vi "main.vi"() -> ()   [LabVIEW 2020]
uses:
  <vilib>/DAQmx/read.llb/DAQmx Read (Analog 1D DBL 1Chan NSamp).vi
  <vilib>/Analysis/baseanly.llb/Mean (DBL).vi
  <vilib>/Utility/file.llb/Write Delimited Spreadsheet (string).vi
  <vilib>/DAQmx/create/channels.llb/DAQmx Create Channel (AI-Current-Basic).vi
  <vilib>/DAQmx/configure/timing.llb/DAQmx Timing (Sample Clock).vi
  <vilib>/DAQmx/create/channels.llb/DAQmx Create Channel (AI-Voltage-Basic).vi
  <vilib>/Utility/file.llb/Write Delimited Spreadsheet (DBL).vi
  <vilib>/DAQmx/miscellaneous.llb/DAQmx Fill In Error Info.vi
  sub_vi/Timing.llb/getRelativeTime(Host).vi
  <vilib>/Analysis/NI_AALBase.lvlib
  sub_vi/Timing.llb/Timing.lvlib
  sub_vi/PlotGraph.llb/GraphPlot.lvlib
panel:
  out "period(hz)":dbl(knob) scale=0.0..30.0
  out "ElapseTime":string
  out "power_value":dbl format="%0.2f"
  in  "FileName":string="power"
  out "power_praph":cluster{dbl[], dbl[]}(graph)
  out "VI_graph":cluster{dbl[], dbl[]}[](graph)
  out "enable_channel":bool
  out "enable_channel":bool
  in  "stop":bool
  out "ampere_value":dbl format="%0.2f"
  out "voltage_value":dbl format="%0.2f"
  out "ampere_graph":dbl[](graph)
  out "voltage_graph":dbl[](graph)
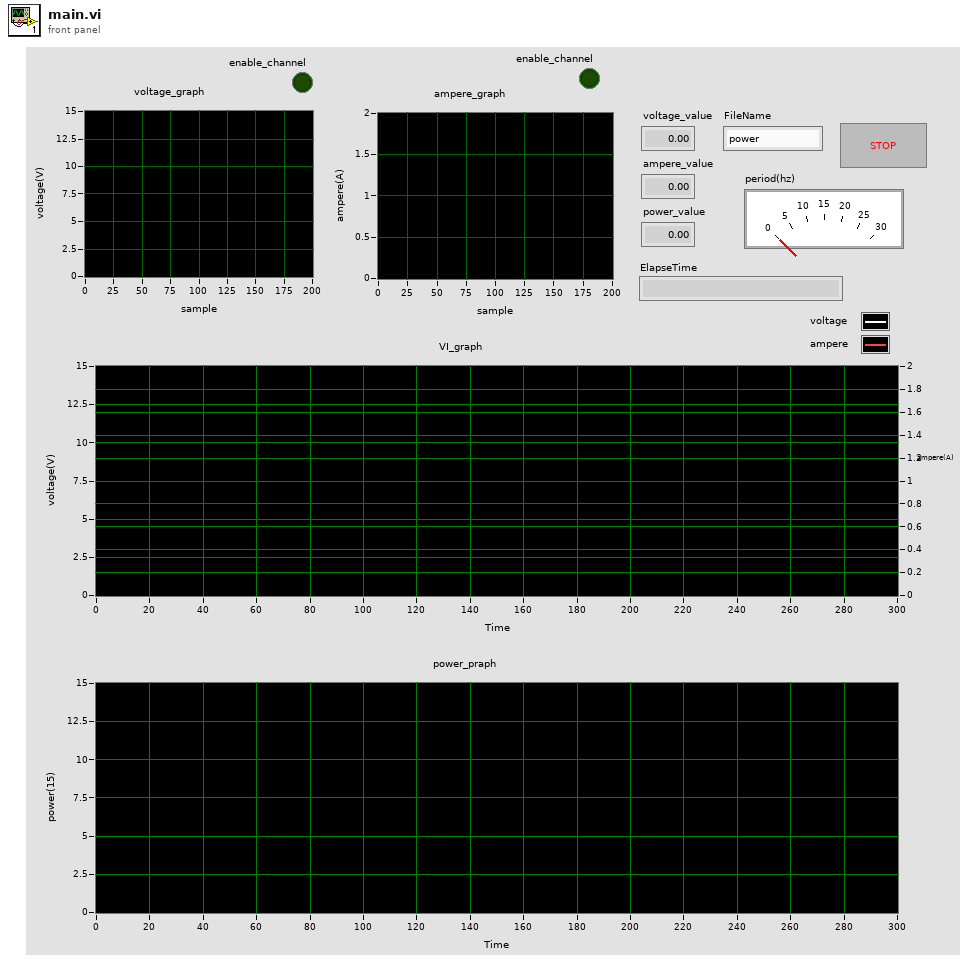
[diagram p1: front panel]
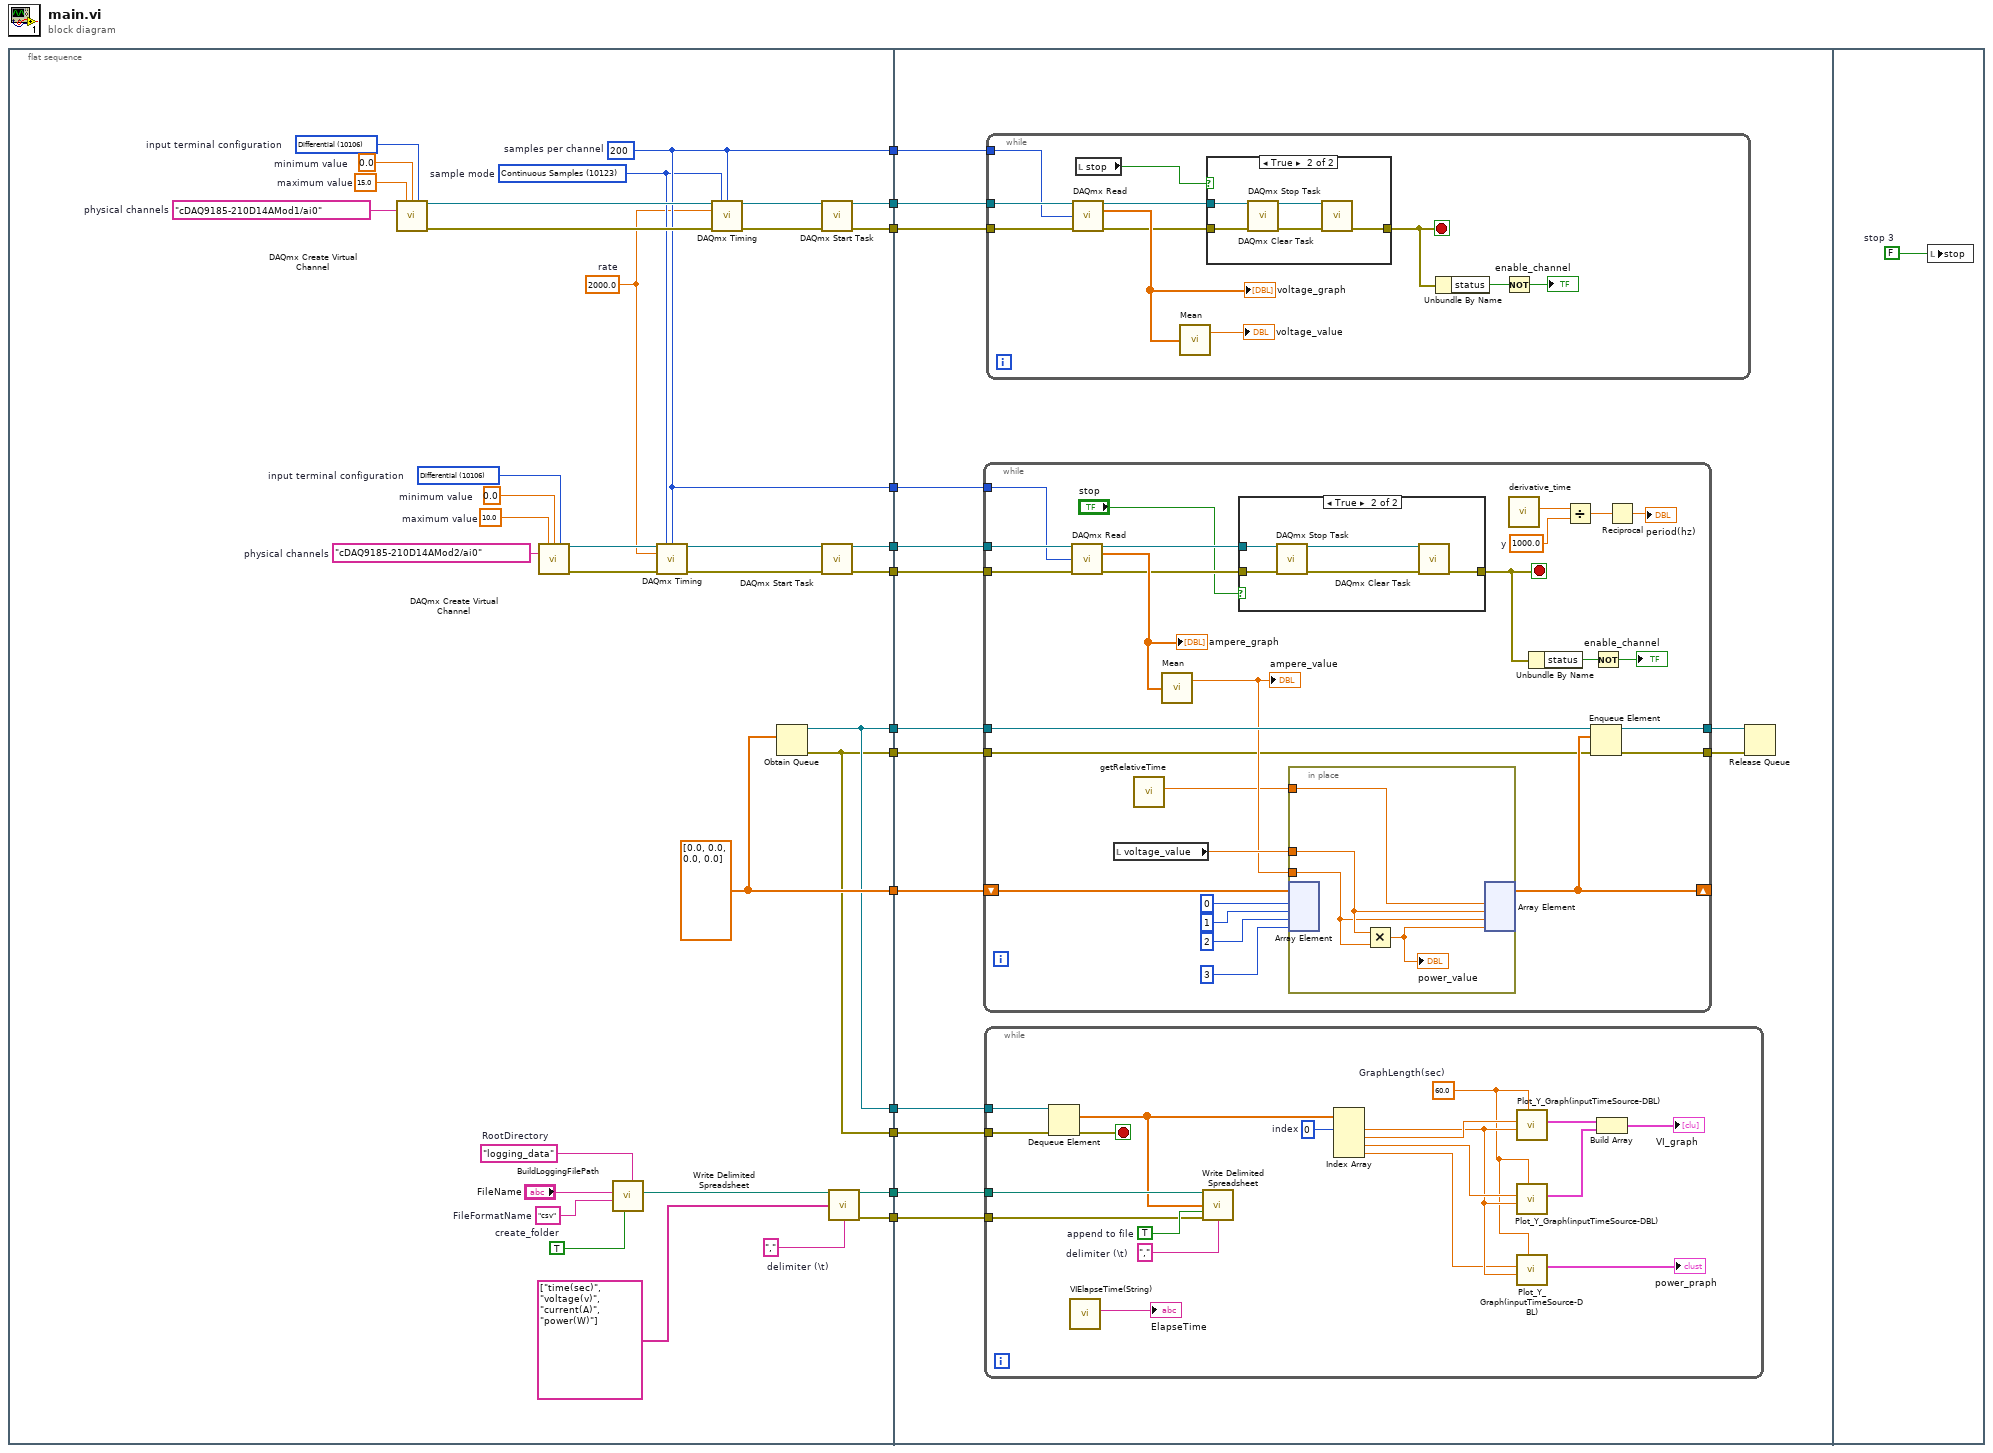
[diagram p0: block diagram]
diagram:
  n1 = flat-sequence {
    tunnel: [w44] -> w13
    tunnel: [w40] -> w12
    tunnel: [w35] -> w11
    tunnel: [w34] -> w10
    tunnel: [w30] -> w9
    tunnel: [w30] -> w8
    tunnel: [w32] -> w7
    tunnel: [w33] -> w6
    tunnel: [w31] -> w5
    tunnel: [w32] -> w4
    tunnel: [w31] -> w3
    tunnel: [w20] -> w2
    tunnel: [w18] -> w1
    tunnel: w13 -> [w63]
    tunnel: w12 -> [w62]
    tunnel: w11 -> [w60]
    tunnel: w10 -> [w59]
    tunnel: w9 -> [w58]
    tunnel: w8 -> [w61]
    tunnel: w7 -> [w57]
    tunnel: w6 -> [w56]
    tunnel: w5 -> [w55]
    tunnel: w4 -> [w54]
    tunnel: w3 -> [w53]
    tunnel: w2 -> [w52]
    tunnel: w1 -> [w51]
    frame #0 {
      w14 = 15.0  # maximum value
      w15 = 0.0  # minimum value
      w16 = 10.0  # maximum value
      w17 = 0.0  # minimum value
      w19 = ","  # delimiter (\t)
      w23 = TRUE  # create_folder
      w24 = "logging_data"  # RootDirectory
      w25 = "csv"  # FileFormatName
      w27 = 10106 items=["Default"=-1, "RSE"=10083, "NRSE"=10078, "Differential"=10106, "Pseudodifferential"=12529]  # input terminal configuration
      w33 = dbl[] [0.0, 0.0, 0.0, 0.0]
      w30 = 200  # samples per channel
      w28 = 2000.0  # rate
      w29 = 10123 items=["Finite Samples"=10178, "Continuous Samples"=10123, "Hardware Timed Single Point"=12522]  # sample mode
      w45 = 10106 items=["default"=-1, "RSE"=10083, "NRSE"=10078, "Differential"=10106, "Pseudodifferential"=12529]  # input terminal configuration
      w47 = tag "cDAQ9185-210D14AMod2/ai0"  # physical channels
      w48 = tag "cDAQ9185-210D14AMod1/ai0"  # physical channels
      n2 = call-poly <vilib>:"DAQmx Create Virtual Channel.vi"("maximum value"=w14, "minimum value"=w15, "input terminal configuration"=w27, "physical channels"=w48) -> ("task out"=w39:refnum<k21>, "error out"=w38:errorcluster)  [unwired: 10 in]
      n3 = call-poly <vilib>:"DAQmx Create Virtual Channel.vi"("maximum value"=w16, "minimum value"=w17, "input terminal configuration"=w45, "physical channels"=w47) -> ("task out"=w43:refnum<k21>, "error out"=w42:errorcluster)  [unwired: 10 in]
      n4 = call "BuildLoggingFilePath.vi"("SubFolderName"=w24, "create_folder"=w23, "FileFormatName"=w25, "FileName"="FileName") -> ("appended path"=w22:path)  [unwired: 7 in]
      n5 = call-poly <vilib>:"DAQmx Timing.vi"("task/channels in"=w43, "sample mode"=w29, "samples per channel"=w30, "rate"=w28, "error in"=w42) -> ("task out"=w46:refnum<k21>, "error out"=w41:errorcluster)  [unwired: 9 in]
      n6 = call-poly <vilib>:"DAQmx Timing.vi"("task/channels in"=w39, "sample mode"=w29, "samples per channel"=w30, "rate"=w28, "error in"=w38) -> ("task out"=w37:refnum<k21>, "error out"=w36:errorcluster)  [unwired: 9 in]
      n7 = Obtain Queue(element data type=w33) -> (queue out=w32:refnum<queue>, error out=w31:errorcluster)  [unwired: 4 in, 1 out]
      n8 = call <vilib>:"DAQmx Start Task.vi"("task/channels in"=w37, "error in"=w36) -> ("task out"=w35:refnum<k21>, "error out"=w34:errorcluster)  [unwired: 12 in]
      n9 = call <vilib>:"DAQmx Start Task.vi"("task/channels in"=w46, "error in"=w41) -> ("task out"=w44:refnum<k21>, "error out"=w40:errorcluster)  [unwired: 12 in]
      n10 = call-poly <vilib>:"Write Delimited Spreadsheet.vi"("file path (dialog if empty)"=w22, "1D data"=string[] ["time(sec)", "voltage(v)", "current(A)", "power(W)"], "delimiter (\\t)"=w19) -> ("new file path (Not A Path if cancelled)"=w20:path, "error out"=w18:errorcluster)  [unwired: 11 in]
    }
    frame #1 {
      n11 = while {
        tunnel: w62 -> [w108]
        tunnel: w61 -> [w107]
        tunnel: w63 -> [w109]
        tunnel: w57 -> [w101]
        shift-right: [w95] -> _
        shift-left: w56 -> [w100]
        tunnel: w55 -> [w94]
        tunnel: [w93] -> w50
        tunnel: [w91] -> w49
        stop <- w89 stop-if-true
        w83 = 1000.0  # y
        n12 = call-poly <vilib>:"DAQmx Read.vi"("task/channels in"=w109, "number of samples per channel"=w107, "error in"=w108) -> ("task out"=w105:refnum<k21>, "data"=w106:dbl[], "error out"=w104:errorcluster)  [unwired: 10 in]
        "ampere_graph" <- w106
        n13 = local read "voltage_value"() -> (w97:dbl)
        n14 = call-poly "getRelativeTime.vi"() -> ("getRelativeTime(sec)"=w90:dbl)  [unwired: 11 in]
        n15 = call-poly <vilib>:"Mean.vi"("X"=w106) -> ("mean"=w96:dbl)  [unwired: 1 out]
        "ampere_value" <- w96
        n16 = case shown="True" "stop" {
          tunnel: w105 -> [_ w119]
          tunnel: w104 -> [w114 w118]
          tunnel: [w114 w116] -> w89
          frame False {
          }
          frame True {
            n17 = call <vilib>:"DAQmx Stop Task.vi"("task/channels in"=w119, "error in"=w118) -> ("task out"=w115:refnum<k21>, "error out"=w117:errorcluster)  [unwired: 12 in]
            n18 = call <vilib>:"DAQmx Clear Task.vi"("task in"=w115, "error in"=w117) -> ("error out"=w116:errorcluster)  [unwired: 13 in]
          }
        }
        n19 = in-place {
          in-place-border: w97 -> [w112]
          in-place-border: w96 -> [w111]
          in-place-border: w90 -> [w113]
          n20 = in-place-array #1(w100, 0, 1, 2, 3) -> ()  [unwired: 4 out]
          n21 = Multiply(x=w112, y=w111) -> (x*y=w110:dbl)
          "power_value" <- w110
          n22 = in-place-array #1(w113, w112, w111, w110) -> (w95:dbl[])  [unwired: 4 out]
        }
        n23 = call "derivative_time.vi"() -> ("derivative_time(msec)"=w86:dbl)  [unwired: 11 in]
        n24 = Unbundle By Name(w89) -> ("status"=w102:bool)
        n25 = Divide(x=w86, y=w83) -> (x/y=w84:dbl)
        n26 = Enqueue Element(queue=w101, element=w95, error in (no error)=w94) -> (queue out=w93:refnum<queue>, error out=w91:errorcluster)  [unwired: 1 in, 1 out]
        n27 = Not(x=w102) -> (.not. x?=→"enable_channel":bool)
        n28 = Reciprocal(x=w84) -> (1/x=→"period(hz)":dbl)
      }
      n29 = while {
        tunnel: w54 -> [w82]
        tunnel: w53 -> [w81]
        tunnel: w52 -> [w80]
        tunnel: w51 -> [w77]
        stop <- w74 stop-if-true
        w65 = 60.0  # GraphLength(sec)
        w72 = 0  # index
        w78 = TRUE  # append to file
        w79 = ","  # delimiter (\t)
        n30 = Dequeue Element(queue=w82, error in (no error)=w81) -> (element=w73:dbl[], error out=w74:errorcluster)  [unwired: 1 in, 2 out]
        n31 = call "VIElapseTime(String).vi"() -> ("ElapseTime"=→"ElapseTime":string)  [unwired: 11 in]
        n32 = call-poly <vilib>:"Write Delimited Spreadsheet.vi"("file path (dialog if empty)"=w80, "1D data"=w73, "append to file? (new file:F)"=w78, "error in (no error)"=w77, "delimiter (\\t)"=w79) -> ()  [unwired: 9 in, 2 out]
        n33 = Index Array "Index Array"(array=w73, index #1=w72) -> (element #1=w67:dbl, element #2=w68:dbl, element #3=w69:dbl, element #4=w66:dbl)  [unwired: 3 in]
        n34 = call "Plot_Y_Graph(inputTimeSource-DBL).vi"("GraphLength(sec)"=w65, "TimeSource"=w67, "DataInput(Y-Value)"=w68) -> ("output_plot"=w76:cluster{dbl[], dbl[]})  [unwired: 8 in]
        n35 = call "Plot_Y_Graph(inputTimeSource-DBL).vi"("GraphLength(sec)"=w65, "TimeSource"=w67, "DataInput(Y-Value)"=w69) -> ("output_plot"=w70:cluster{dbl[], dbl[]})  [unwired: 8 in]
        n36 = call "Plot_Y_Graph(inputTimeSource-DBL).vi"("GraphLength(sec)"=w65, "TimeSource"=w67, "DataInput(Y-Value)"=w66) -> ("output_plot"=→"power_praph":cluster{dbl[], dbl[]})  [unwired: 8 in]
        n37 = Build Array(w76, w70) -> (→"VI_graph":cluster{dbl[], dbl[]}[])
      }
      n38 = while {
        tunnel: w59 -> [w129]
        tunnel: w58 -> [w128]
        tunnel: w60 -> [w130]
        stop <- w122 stop-if-true
        n39 = call-poly <vilib>:"DAQmx Read.vi"("task/channels in"=w130, "number of samples per channel"=w128, "error in"=w129) -> ("task out"=w125:refnum<k21>, "data"=w127:dbl[], "error out"=w124:errorcluster)  [unwired: 10 in]
        "voltage_graph" <- w127
        n40 = local read "stop"() -> (w123:bool)
        n41 = call-poly <vilib>:"Mean.vi"("X"=w127) -> ("mean"=→"voltage_value":dbl)  [unwired: 1 out]
        n42 = case shown="True" w123 {
          tunnel: w125 -> [_ w136]
          tunnel: w124 -> [w131 w135]
          tunnel: [w131 w133] -> w122
          frame False {
          }
          frame True {
            n43 = call <vilib>:"DAQmx Stop Task.vi"("task/channels in"=w136, "error in"=w135) -> ("task out"=w132:refnum<k21>, "error out"=w134:errorcluster)  [unwired: 12 in]
            n44 = call <vilib>:"DAQmx Clear Task.vi"("task in"=w132, "error in"=w134) -> ("error out"=w133:errorcluster)  [unwired: 13 in]
          }
        }
        n45 = Unbundle By Name(w122) -> ("status"=w121:bool)
        n46 = Not(x=w121) -> (.not. x?=→"enable_channel":bool)
      }
      n47 = Release Queue(queue=w50, error in (no error)=w49) -> ()  [unwired: 1 in, 3 out]
    }
    frame #2 {
      w137 = FALSE  # stop 3
      n48 = local write "stop"(w137) -> ()
    }
  }
